vi "Read Raw UTF-8 String.vi"(9 "UTF-8 String":refnum<class "UTF-8 String.lvclass">) -> (1 "Raw UTF-8 String":T1)   [LabVIEW 2020, in "G-Unicode.lvlib" / "UTF-8 String.lvclass"]
doc: "Get the UTF-8 encoded string as a LabVIEW string."
uses:
  UTF-8 String.lvclass
  Raw UTF-8 String.ctl
  UTF-8 String.lvclass/UTF-8 String.ctl
  G-Unicode.lvlib
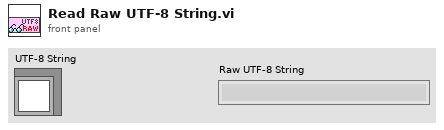
[diagram p1: front panel]
types:
  T1 = typedef "G-Unicode.lvlib/Raw UTF-8 String.ctl" = string
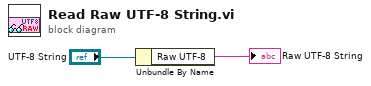
[diagram p0: block diagram]
diagram:
  n1 = Unbundle By Name("UTF-8 String") -> ("Raw UTF-8"=→"Raw UTF-8 String":T1)
